vi "NI VeriStand - Get Event Refnum.vi"(8 "error in (no error)":errorcluster) -> (0 "error out":errorcluster, 3 "Event Ref":refnum<user-event>)   [LabVIEW 2020, in "Custom Device API.lvlib"]
doc: "Returns a registered event refnum that the custom device Configuration VI, which is called when a user instantiates a new instance of a custom device, uses to respond to <B>System Explorer</B> window events."
uses:
  <vilib>/NI VeriStand/Custom Device API/Custom Device API.lvlib
  62ac00c8-7fb5-43b2-9e3e-01ec0adae5ef.vi
  <vilib>/NI VeriStand/Custom Device API/Custom Device Offline Path.vi
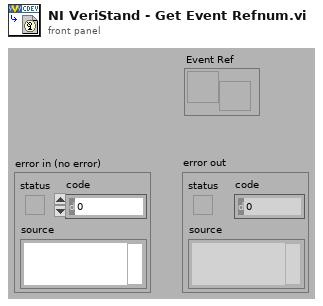
[diagram p1: front panel]
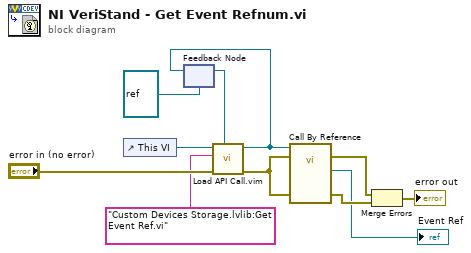
[diagram p0: block diagram]
diagram:
  n1 = control-ref of="This VI"() -> (w3:refnum<vi>)
  n2 = feedback #1(refnum<vi> refnum ("type specifier VI Refnum (for type only)")) -> (w8:refnum<vi>)
  n3 = call "Load API Call.vim"("VI reference in"=w8, "error in (no error)"="error in (no error)", "VI qualified name"="Custom Devices Storage.lvlib:Get Event Ref.vi", "Caller VI ref"=w3) -> ("error out"=w4:errorcluster, "VI reference"=w7:refnum<vi>)  [unwired: 6 in]
  n4 = feedback-in #1(w7) -> ()
  n5 = call-by-ref "?"(reference=w7, error in=w4, 8:"error in (no error)"=w4) -> (error out=w1:errorcluster, 0:"error out"=w11:errorcluster, "Communication"=→"Event Ref":refnum<user-event>)  [unwired: 9 in, 1 out]
  n6 = Merge Errors(w1, w11) -> (→"error out":errorcluster)
